vi "LabVIEWInterface.vi"() -> ()   [LabVIEW 2020]
doc: "DHT11 Temperature and Humidity Sensor\n\nThis example demonstrates how to read the DHT11 sensor included in the LabVIEW Interactions Parts Kit. Make sure\nthat you are using the correct firmware version so the DHT functions are supported. \n\nInstructions:\n1. Select the COM Port associated with the LINX device\n2. Enter the DHT Data Pin\n3. Click the Run Arrow."
uses:
  <vilib>/MakerHub/LINX/Public/Peripherals/Digital/Digital Write 1 Chan.vi
  <vilib>/MakerHub/LINX/Public/Peripherals/Digital/Digital Write N Chans.vi
  <vilib>/MakerHub/LINX/Private/Local IO/LinxDigitalWrite.vi
  <vilib>/MakerHub/LINX/Public/Utilities/Check Channel.vi
  <vilib>/MakerHub/LINX/Public/Utilities/Open Serial.vi
  <vilib>/MakerHub/LINX/Private/Utilties/Generate Error.vi
  <vilib>/MakerHub/LINX/LMH-LINX.lvlib
  <vilib>/MakerHub/LINX/Public/Sensors/Digilent/Interaction Parts Kit/Interaction Parts Kit.lvlib
panel:
  out "Humidity":u8
  in  "Fan Control":bool
  out "Temp (C)":u8(slide) scale=0.0..100.0
  out "Humidity":u8(graph)
  out "Status":bool
  in  "Temp Limit":u8
  in  "Humidity Limit":u8
  in  "Fan Pin":u8
  in  "DHT Data Pin":u8=2
  out "Loop Rate (Hz)":u32
  in  "Serial Port":refnum<visa-resource-name>="COM6"
  in  "Stop Button":bool
  # "Medication storage system"
  # "Config"
  # "Settings"
  # "Environment Status"
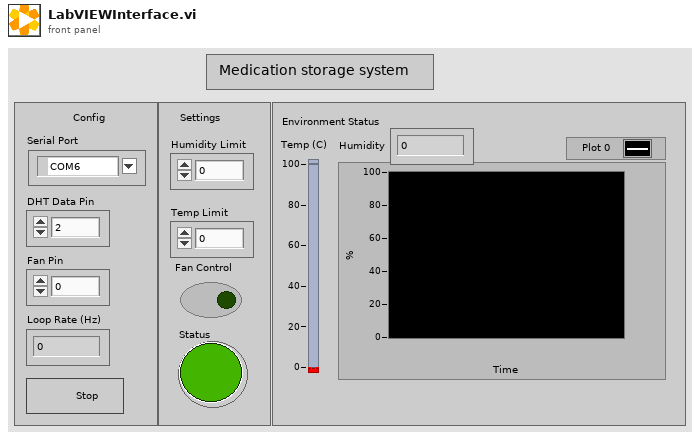
[diagram p1: front panel]
types:
  T1 = typedef "LMH-LINX.lvlib/LINX Ref.ctl" = cluster{"IO":T2, "Interface":T3, "LINX Device Config":T4}
  T2 = typedef "LMH-LINX.lvlib/Platform.ctl" = enum16{"Remote", "Local"}
  T3 = typedef "LMH-LINX.lvlib/Interface.ctl" = enum16{"Serial", "TCP"}
  T4 = typedef "LMH-LINX.lvlib/Device.lvlib/LINX Device Config.ctl" = cluster{"Interface":T3, "COM Port":refnum<visa-resource-name>, "TCP Configuration":T5, "Device Family":u8, "Device ID":u8, "Device Name":string, "TCP Ref":refnum<k5>, "Channels":T6}
  T5 = typedef "LMH-LINX.lvlib/Device.lvlib/TCP Config.ctl" = cluster{"IP Address":string, "Port":u16}
  T6 = typedef "LMH-LINX.lvlib/Channels.ctl" = cluster{"DI":u8[], "DO":u8[], "AI":u8[], "AO":u8[], "PWM":u8[], "QE":u8[], "UART":u8[], "I2C 2":u8[], "SPI":u8[], "CAN":u8[], "Servo":u8[], "AI Ref (V)":dbl, "AI Resolution (Bits)":u8, "AO Ref (V)":dbl, "AO Resolution (Bits)":u8}
  T7 = enum16{"big-endian, network order", "native, host order", "little-endian"}
  T8 = cluster{"Humidity":u8, "Temp (C)":u8, "Temp (F)":u8, "Heat Index (C)":u8, "Heat Index (F)":u8}
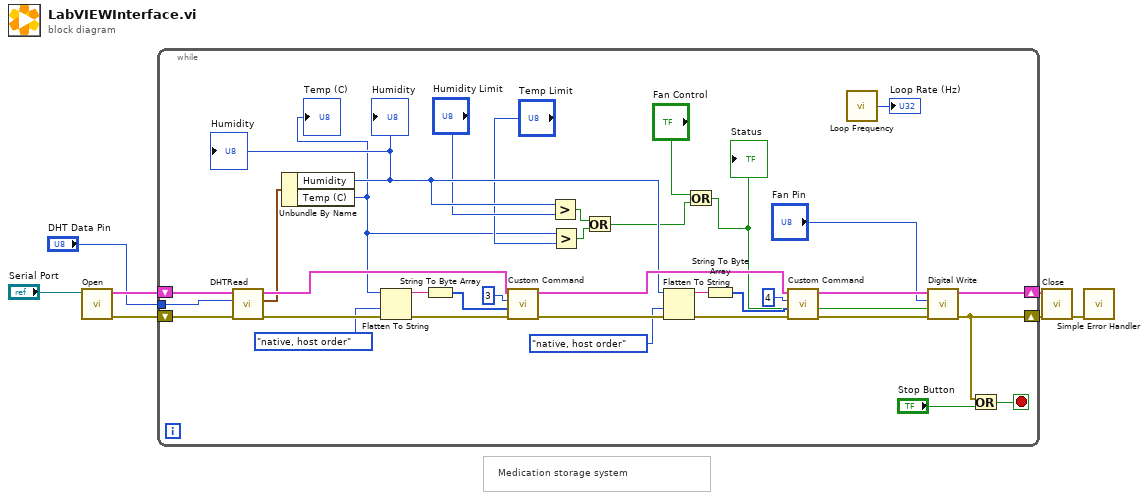
[diagram p0: block diagram]
diagram:
  # "Medication storage system"
  n1 = call-poly <vilib>:"Open.vi"("Serial Port"="Serial Port") -> ("Error Out"=w6:errorcluster, "LINX Resource"=w7:T1)  [unwired: 8 in, 1 out]
  n2 = while {
    shift-right: [w19] -> w5
    shift-left: w7 -> [w42]
    shift-right: [w18] -> w4
    shift-left: w6 -> [w41]
    tunnel: "DHT Data Pin" -> [w37]
    stop <- w39 stop-if-true
    n3 = call <vilib>:"DHTRead.vi"("Error In"=w41, "DHT Data Pin"=w37, "LINX Resource"=w42) -> ("Error Out"=w28:errorcluster, "DHT Readings"=w23:T8, "LINX Resource"=w36:T1)  [unwired: 6 in]
    n4 = Unbundle By Name(w23) -> ("Humidity"=w16:u8, "Temp (C)"=w11:u8)
    "Humidity" <- w16
    "Temp (C)" <- w11
    "Humidity" <- w16
    n5 = Flatten To String(anything=w11, byte order (0:big-endian, network order)=T7."native, host order", error in (no error)=w28) -> (data string=w30:string, error out=w27:errorcluster)  [unwired: 1 in, 1 out]
    n6 = String To Byte Array(string=w30) -> (unsigned byte array=w31:u8[])
    n7 = call <vilib>:"Custom Command.vi"("Error In"=w27, "Data"=w31, "Custom Command Number"=u16 3, "LINX Resource"=w36) -> ("Error Out"=w26:errorcluster, "LINX Resource"=w34:T1)  [unwired: 4 in, 2 out]
    n8 = Greater?(x=w16, y="Humidity Limit") -> (0:w13:bool)
    n9 = Greater?(x=w11, y="Temp Limit") -> (0:w12:bool)
    n10 = Or(x=w13, y=w12) -> (x .or. y?=w9:bool)
    n11 = Flatten To String(anything=w16, byte order (0:big-endian, network order)=T7."native, host order", error in (no error)=w26) -> (data string=w29:string, error out=w25:errorcluster)  [unwired: 1 in, 1 out]
    n12 = Or(x="Fan Control", y=w9) -> (x .or. y?=w8:bool)
    "Status" <- w8
    n13 = String To Byte Array(string=w29) -> (unsigned byte array=w32:u8[])
    n14 = call <vilib>:"Custom Command.vi"("Error In"=w25, "Data"=w32, "Custom Command Number"=u16 4, "LINX Resource"=w34) -> ("Error Out"=w20:errorcluster, "LINX Resource"=w21:T1)  [unwired: 4 in, 2 out]
    n15 = call <vilib>:"Loop Frequency.vi"() -> ("Loop Rate (Hz)"=→"Loop Rate (Hz)":u32)
    n16 = call-poly <vilib>:"Digital Write.vi"("Error In"=w20, "Output Value"=w8, "DO Channel"="Fan Pin", "LINX Resource"=w21) -> ("Error Out"=w18:errorcluster, "LINX Resource"=w19:T1)  [unwired: 6 in]
    n17 = Or(x=w18, y="Stop Button") -> (x .or. y?=w39:bool)
  }
  n18 = call <vilib>:"Close.vi"("Error In"=w4, "LINX Resource"=w5) -> ("Error Out"=w1:errorcluster)  [unwired: 9 in]
  n19 = call <vilib>:"Simple Error Handler.vi"("error in (no error)"=w1) -> ()  [unwired: 4 in, 5 out]
